vi "Pre-Actor.vi"(8 "error in (no error)":errorcluster, 11 "AnalogInput in":refnum<class "AnalogInput.lvclass">) -> (0 "error out":errorcluster, 3 "AnalogInput out":refnum<class "AnalogInput.lvclass">)   [LabVIEW 2019, in "AnalogInput.lvlib" / "AnalogInput.lvclass"]
doc: "This override VI is to provide the means for children classes to perform application specific post launch initialization functions that must be performed *prior* to calling the actor."
uses:
  Library/AnalogInput.lvclass
  builds/Engine/Engine.lvlibp/Project/Engine.lvclass
  C:/Users/Public/Documents/Development/builds/Engine/Engine.lvlibp/Project/Engine.lvclass
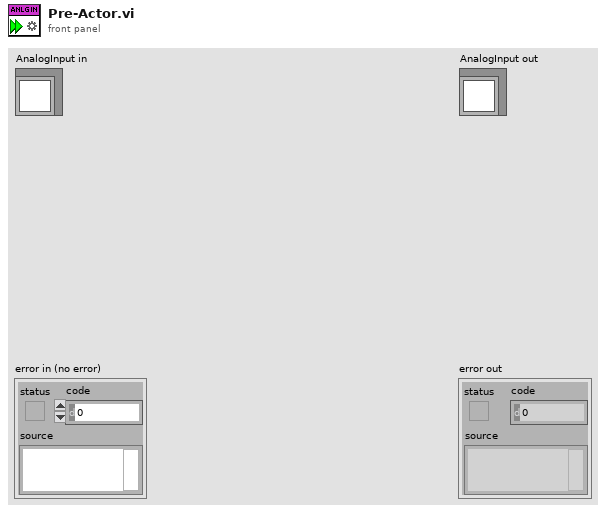
[diagram p1: front panel]
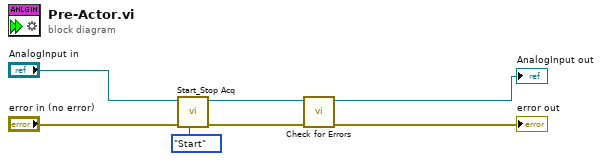
[diagram p0: block diagram]
diagram:
  n1 = call-dynamic "Start_Stop Acq.vi"("Start/Stop"=enum16{"Start", "Stop"}."Start", "error in (no error)"="error in (no error)", "AnalogInput in"="AnalogInput in") -> ("error out"=w3:errorcluster, "AnalogInput out"=w4:refnum<class "AnalogInput.lvclass">)  [unwired: 7 in]
  n2 = call "Check for Errors.vi"("error in"=w3, "Engine in"=w4) -> ("error out"=→"error out":errorcluster, "Engine out"=→"AnalogInput out":refnum<class "AnalogInput.lvclass">)  [unwired: 8 in]
